vi "sabertooth packetized v2 set settings.vi"() -> ()   [LabVIEW 2018]
uses:
  package/controls/Sabertooth Address Select.ctl
  package/controls/Sabertooth Command Select.ctl
  package/controls/Sabertooth Baud Rate Select.ctl
  <vilib>/Instr/_visa.llb/VISA Configure Serial Port (Instr).vi
panel:
  in  "Current Baud Rate":T1=115200 items=["2400 baud"=2400, "9600 baud"=9600, "19200 baud"=19200, "38400 baud"=38400, "115200 baud"=115200]
  in  "Data":u32
  in  "Command List":T2=15 items=["Min voltage"=2, "Max voltage"=3, "Serial Timeout"=14, "Baud Rate"=15, "Ramping"=16, "Deadband"=17]
  in  "Sabertooth Addresses":T3=129 items=["Sabertooth 1"=128, "Sabertooth 2"=129, "Sabertooth 3"=130, "Sabertooth 4"=131, "Sabertooth 5"=132, "Sabertooth 6"=133, "Sabertooth 7"=134, "Sabertooth 8"=135]
  # "Setting Commands Data from Sabertooth datasheet: https://www.dimensionengineering.com/datasheets/Sabertooth2x60.pdf\n\n\n\nCommands are already in menu ring \"Command List\"\n<-\n\n2: Min voltage (decimal 2, binary 0b00000010, hex 0h02)\nThis is used to set a custom minimum voltage for the battery feeding the Sabertooth. If the\nbattery voltage drops below this value, the output will shut down. This value is cleared at startup,\nso much be set each run. The value is sent in .2 volt increments with a command of zero\ncorresponding to 6v, which is the minimum. Valid data is from 0 to 120. The function for\nconverting volts to command data is\nValue = (desired volts-6) x 5\n\n3: Max voltage (decimal 3, binary 0b0000011, hex 0h03)\nThis is used to set a custom maximum voltage. If you are using a power supply that cannot sink\ncurrent such as an ATX supply, the input voltage will rise when the driver is regenerating\n(slowing down the motor) Many ATX type supplies will shut down if the output voltage on the\n12v supply rises beyond 16v. If the driver detects an input voltage above the set limit, it will put\nthe motor into a hard brake until the voltage drops below the set point again. This is inefficient,\nbecause the energy is heating the motor instead of recharging a battery, but may be necessary.\nThe driver comes preset for a maximum voltage of 30V. The range for a custom maximum\nvoltage is 0v-25v. The formula for setting a custom maximum voltage is\nValue = Desired Volts*5.12\nIf you are using any sort of battery, then this is not a problem and the max voltage should be left\nat the startup default. \n\n14: Serial Timeout (decimal 14, binary 0b00001110, hex 0h0e)\nThis setting determines how long it takes for the motor driver to shut off if it has not received a\ncommand recently. Serial Timeout is off by default. A command of 0 will disable the timeout if\nyou had previously enabled it. The timeout scales 1 unit per 100ms of timeout, so a command of\n10 would make a timeout of 1000ms. This setting does not persist through a power cycle or in\nany mode other than packet Serial.\n\n15: Baud Rate (decimal 15, binary 0b00001111, hex 0h0f)\nThis value remains until it is changed and does persist through a power cycle. The values are:\n1: 2400 baud\n2: 9600 baud (default)\n3: 19200 baud\n4: 38400 baud\n5: 115200 baud\n\n16: Ramping (decimal 16, binary 0b00010000, hex 0h10)\nThis adjusts or disables the ramping feature found on the Sabertooth 2x60. This adjustment\napplies to all modes, even R/C and analog mode. Values between 1 and 10 are Fast Ramp;\nvalues between 11 and 20 are Slow Ramp; values between 21 and 80 are Intermediate Ramp.\nFast Ramping is a ramp time of 256/(~1000xCommand value). Ramp time is the delay between\nfull forward and full reverse speed.\n1: 1/4 second ramp (default)\n2: 1/8 second ramp\n3: 1/12 second ramp\nSlow and Intermediate Ramping are a ramp time of 256/[15.25x(Command value – 10)]\nSee Figures 8.1 and 8.2 in the Appendix for a graph of values.\n\n17: Deadband (decimal 17, binary 0b00010001, hex 0h11)\nThis determines the extent of the Sabertooth’s deadband – the range of commands close to\n“stop” that will be interpreted as stop. This setting applies to all modes and persists through a\npower cycle. The commands range from 0 to 127 and the formula is as follows:\n127-command < motors off < 128+command\nThus, a command of 3 would shut the motors off with speed commands between 124 and 131.\nA command of 0 sets the deadband to its default, which is 124 < off < 131 in serial mode."
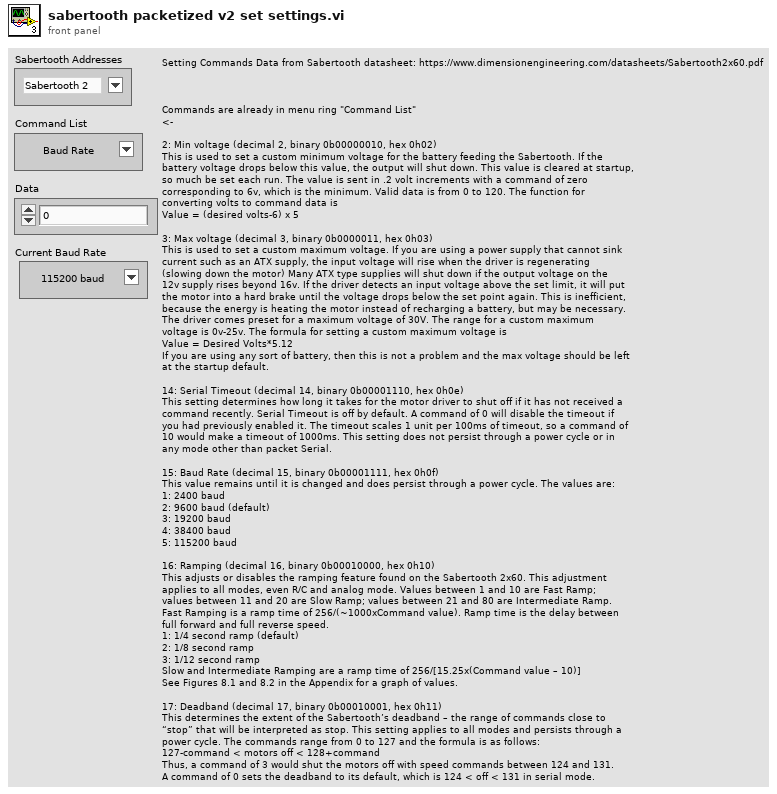
[diagram p1: front panel]
types:
  T1 = typedef "Sabertooth Baud Rate Select.ctl" = u32
  T2 = typedef "Sabertooth Command Select.ctl" = u8
  T3 = typedef "Sabertooth Address Select.ctl" = u8
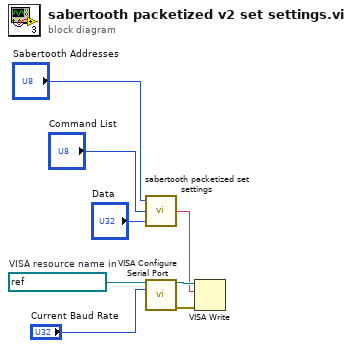
[diagram p0: block diagram]
diagram:
  w8 = refnum<visa-resource-name> "ASRL1::INSTR"  # VISA resource name in
  n1 = call "sabertooth packetized set settings.vi"("Data"="Data", "Command List"="Command List", "Sabertooth Addresses"="Sabertooth Addresses") -> ("msg out"=w5:string)
  n2 = call-poly "VISA Configure Serial Port"("VISA resource name"=w8, "baud rate (9600)"="Current Baud Rate") -> ("VISA resource name out"=w7:refnum<visa-resource-name>, "error out"=w6:errorcluster)  [unwired: 12 in]
  n3 = VISA Write(VISA resource name=w7, write buffer=w5, error in (no error)=w6) -> ()  [unwired: 3 out]
